vi "setPaths.vi"(0 "reference in":refnum<class "File Controller.lvclass">, 5 "filePaths":path[](array[path]), 7 "outlookTemplatePaths":path[](array[path]), 9 "attachmentTemplatePaths":path[](array[path]), 11 "error in (no error)":errorcluster) -> (4 "reference out":refnum<class "File Controller.lvclass">, 15 "error out":errorcluster)   [LabVIEW 2015, in "File Controller.lvclass"]
uses:
  File Controller.lvclass
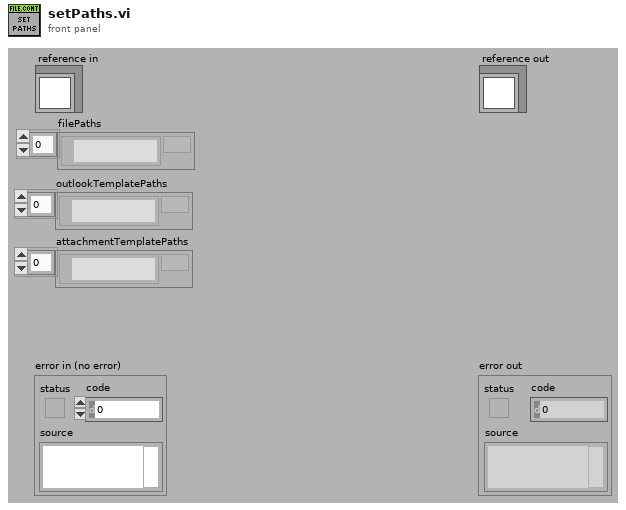
[diagram p1: front panel]
types:
  T1 = typedef "File Controller.lvclass/ObjectAttributesRef.ctl" = refnum<data-value>
  T2 = typedef "File Controller.lvclass/ObjectAttributes.ctl" = cluster{"MyAttribute":dbl, "excelFile_refs":refnum<class "excelFile.lvclass">[], "filePaths":path[], "outlookTemplatePaths":path[], "attachmentTemplatePaths":path[], "configFilePath":path, "not_setting":bool[], "python_ref":refnum<class "python.lvclass">}
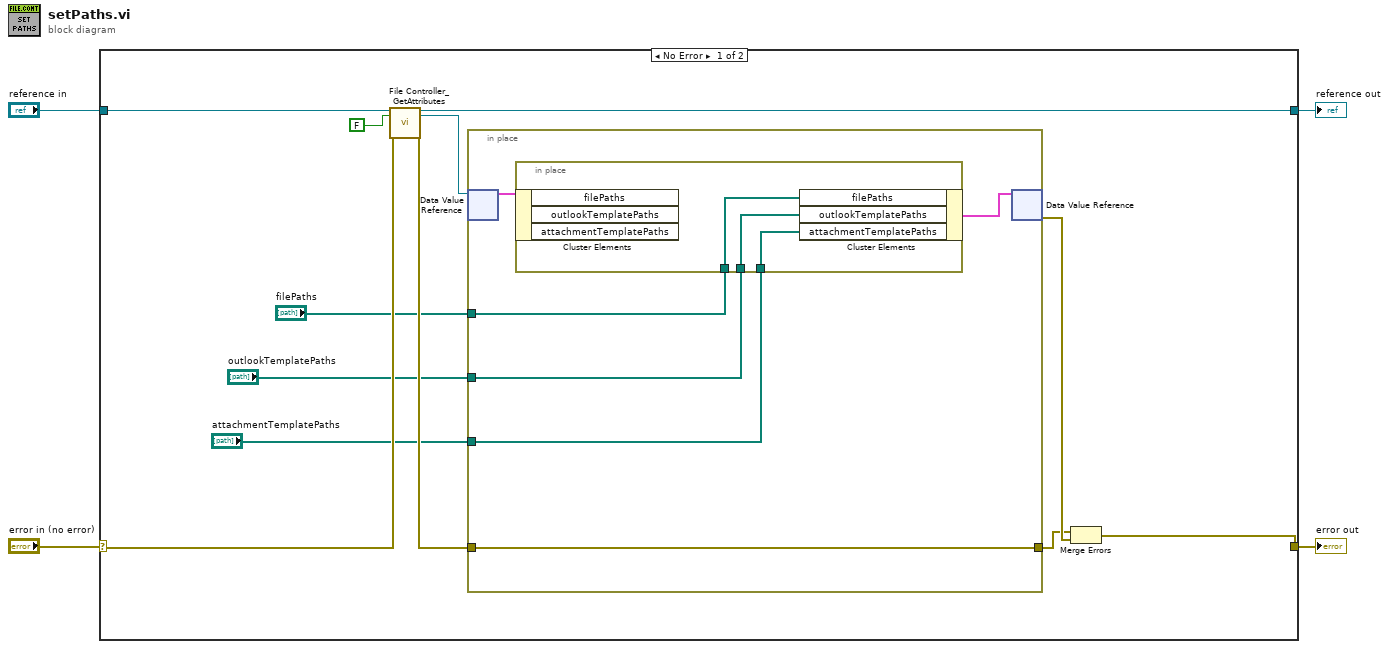
[diagram p0: block diagram]
diagram:
  n1 = case shown="No Error" "error in (no error)" {
    selector: "error in (no error)" -> [w11 w27]
    tunnel: [w16 w27] -> w3
    tunnel: [w9 w26] -> w1
    tunnel: "reference in" -> [w13 w26]
    frame No Error {
      n2 = call "File Controller_GetAttributes.vi"("reference in"=w13, "return data? (T)"=FALSE, "error in (no error)"=w11) -> ("reference out"=w9:refnum<class "File Controller.lvclass">, "attributes ref"=w8:T1, "error out"=w10:errorcluster)  [unwired: 13 in, 1 out]
      n3 = in-place {
        in-place-border: w10 -> [w20]
        in-place-border: [w20] -> w14
        in-place-border: "filePaths" -> [w19]
        in-place-border: "outlookTemplatePaths" -> [w18]
        in-place-border: "attachmentTemplatePaths" -> [w17]
        n4 = in-place-dvr #1(w8) -> (w21:T2)  [unwired: 1 out]
        n5 = in-place {
          in-place-border: w19 -> [w25]
          in-place-border: w18 -> [w24]
          in-place-border: w17 -> [w23]
          n6 = in-place-cluster #2(w21) -> ()  [unwired: 3 out]
          n7 = in-place-cluster #2("filePaths"=w25, "outlookTemplatePaths"=w24, "attachmentTemplatePaths"=w23) -> (w22:T2)
        }
        n8 = in-place-dvr #1(w22) -> (w15:errorcluster)  [unwired: 1 out]
      }
      n9 = Merge Errors(w14, w15) -> (w16:errorcluster)
    }
    frame Error {
    }
  }
  "error out" <- w3
  "reference out" <- w1
